vi "New Items (inline).vi"(8 "error in (no error)":errorcluster, 10 "New Items":refnum<class "BetterItem.lvclass">[](array[class]), 11 "BetterHandle in":refnum<class "BetterHandle.lvclass">) -> (0 "error out":errorcluster, 3 "BetterHandle out":refnum<class "BetterHandle.lvclass">)   [LabVIEW 2020, in "BetterDragAndDrop.lvlib" / "BetterHandle.lvclass"]
uses:
  BetterHandle.lvclass
  BetterTreeItem/BetterItem.lvclass
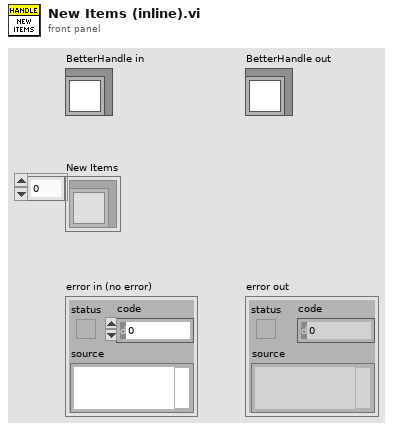
[diagram p1: front panel]
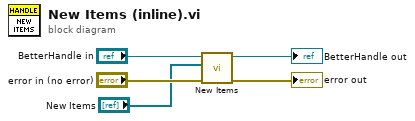
[diagram p0: block diagram]
diagram:
  n1 = call-dynamic "New Items.vi"("error in (no error)"="error in (no error)", "New Items"="New Items", "BetterHandle in"="BetterHandle in") -> ("error out"=→"error out":errorcluster, "BetterHandle out"=→"BetterHandle out":refnum<class "BetterHandle.lvclass">)  [unwired: 7 in]
